vi "Three Ball-Copy (Warning I, Carter did this).vi"() -> ()   [LabVIEW 2014]
uses:
  Team Code/Robot Global Data.vi
panel:
  in  "milliseconds to wait to pull in second ball":u32=1000
  out "Angle":dbl
  out "Distance (in)":dbl
  in  "Min. Power":dbl=0.1 format="%#_13g"
  in  "Roller / Drive Ratio":dbl=1.0
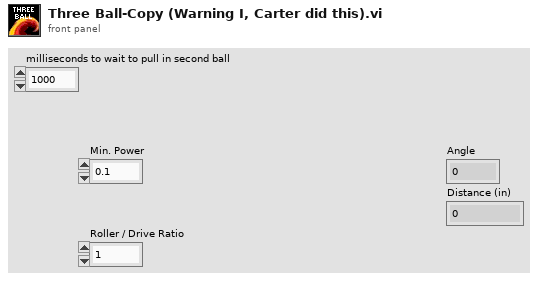
[diagram p1: front panel]
types:
  T1 = cluster{"FIRE!!!":bool, "Loader":bool, "Lock":bool, "Load":bool, "Pass":bool, "Grab":bool, "PANIC":bool, "Don't Cock":bool, "Roller Speed":dbl}
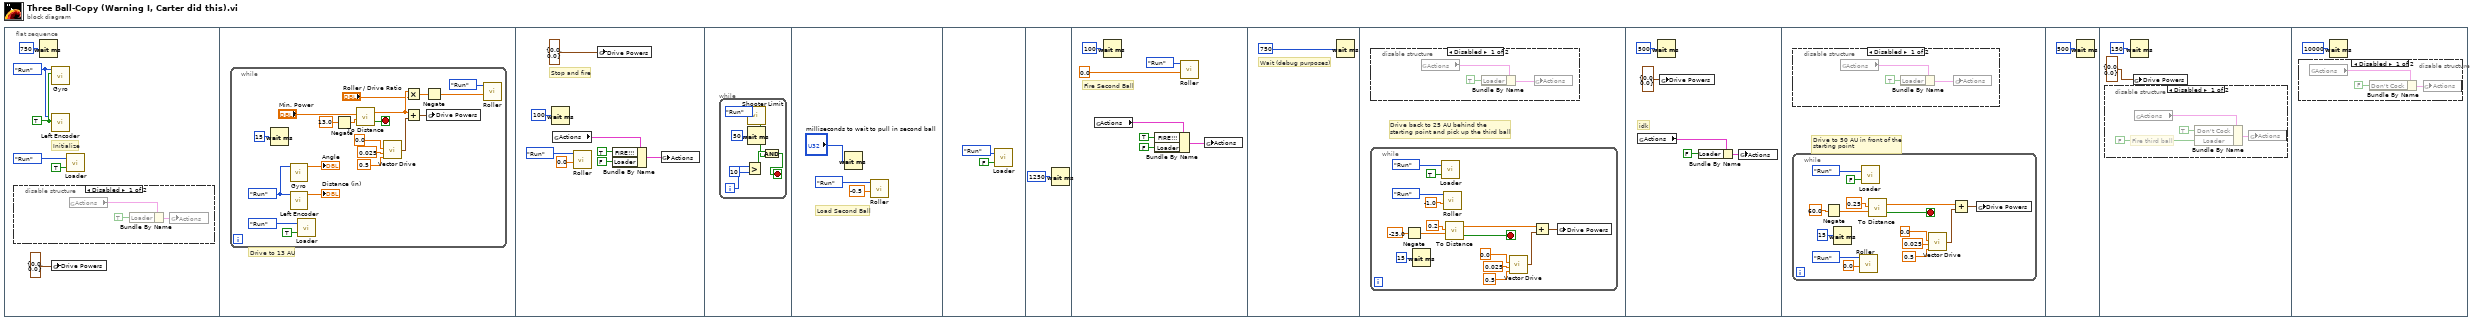
[diagram p0: block diagram]
diagram:
  n1 = flat-sequence {
    frame #0 {
      w5 = enum16{"Start", "Run", "End"}."Run" ("Enum")
      w6 = TRUE ("Reset")
      # "Initialize"
      n2 = disable-structure shown="Disabled" {
        frame Disabled {
          n3 = global read "Robot Global Data.vi" "Actions"() -> (w8:T1)
          n4 = Bundle By Name(cluster=w8, "Loader"=TRUE ("Primary Action")) -> (w9:T1)
          n5 = global write "Robot Global Data.vi" "Actions"(w9) -> ()
        }
        frame Enabled {
        }
      }
      n6 = Wait (ms)(milliseconds to wait=u32 750) -> ()  [unwired: 1 out]
      n7 = call "Gyro.vi"("Reset"=w6, "Enum"=w5) -> ()  [unwired: 9 in, 1 out]
      n8 = call "Left Encoder.vi"("Reset"=w6, "Enum"=w5) -> ()  [unwired: 8 in, 2 out]
      n9 = global write "Robot Global Data.vi" "Drive Powers"(cluster{"Right":dbl, "Left":dbl} {"Right"=0.0, "Left"=0.0} ("Drive Powers")) -> ()
      n10 = call "Loader.vi"("Down (Forward)"=TRUE, "Enum"=enum16{"Start", "Run", "End"}."Run") -> ()  [unwired: 1 out]
    }
    frame #1 {
      # "Drive to 13 AU"
      n11 = while {
        stop <- w28 stop-if-true
        w21 = enum16{"Start", "Run", "End"}."Run" ("Enum")
        n12 = Wait (ms)(milliseconds to wait=u32 15) -> ()  [unwired: 1 out]
        n13 = call "Gyro.vi"("Enum"=w21) -> ("Angle"=→"Angle":dbl)  [unwired: 10 in]
        n14 = call "Left Encoder.vi"("Enum"=w21) -> ("Distance (in)"=→"Distance (in)":dbl)  [unwired: 9 in, 1 out]
        n15 = call "Loader.vi"("Down (Forward)"=TRUE, "Enum"=enum16{"Start", "Run", "End"}."Run") -> ()  [unwired: 1 out]
        n16 = Negate(x=13.0) -> (-x=w19:dbl)
        n17 = call "To Distance.vi"("Destination Dist (in)"=w19, "Min. Power"="Min. Power") -> ("Reached Distance"=w28:bool, "Base Speed"=w17:dbl)  [unwired: 2 in]
        n18 = call "Vector Drive.vi"("Tolerance"=0.5, "Min. Power"=0.025, "Angle"=0.0) -> ("Motor Powers"=w24:cluster{"RMotor":dbl, "LMotor":dbl})  [unwired: 1 in]
        n19 = Multiply(x=w17, y="Roller / Drive Ratio") -> (x*y=w14:dbl)
        n20 = Add(x=w17, y=w24) -> (x+y=w23:cluster{"RMotor":dbl, "LMotor":dbl})
        n21 = Negate(x=w14) -> (-x=w13:dbl)
        n22 = global write "Robot Global Data.vi" "Drive Powers"(w23) -> ()
        n23 = call "Roller.vi"("Power"=w13, "Enum"=enum16{"Start", "Run", "End"}."Run") -> ()  [unwired: 2 in]
      }
    }
    frame #2 {
      # "Stop and fire"
      n24 = Wait (ms)(milliseconds to wait=u32 100) -> ()  [unwired: 1 out]
      n25 = global read "Robot Global Data.vi" "Actions"() -> (w36:T1)
      n26 = call "Roller.vi"("Power"=0.0, "Enum"=enum16{"Start", "Run", "End"}."Run") -> ()  [unwired: 2 in]
      n27 = global write "Robot Global Data.vi" "Drive Powers"(cluster{"Right":dbl, "Left":dbl} {"Right"=0.0, "Left"=0.0} ("Drive Powers")) -> ()
      n28 = Bundle By Name(cluster=w36, "FIRE!!!"=TRUE ("Primary Action"), "Loader"=FALSE) -> (w37:T1)
      n29 = global write "Robot Global Data.vi" "Actions"(w37) -> ()
    }
    frame #3 {
      n30 = while {
        i -> [w42]
        stop <- w38 stop-if-true
        n31 = Greater?(x=w42, y=10) -> (0:w40:bool)
        n32 = call "Shooter Limit.vi"("Enum"=enum16{"Start", "Run", "End"}."Run") -> ("Value"=w39:bool)  [unwired: 1 in]
        n33 = Wait (ms)(milliseconds to wait=u32 50) -> ()  [unwired: 1 out]
        n34 = And(x=w40, y=w39) -> (x .and. y?=w38:bool)
      }
    }
    frame #4 {
      # "Load Second Ball"
      n35 = Wait (ms)(milliseconds to wait="milliseconds to wait to pull in second ball") -> ()  [unwired: 1 out]
      n36 = call "Roller.vi"("Power"=-0.5, "Enum"=enum16{"Start", "Run", "End"}."Run") -> ()  [unwired: 2 in]
    }
    frame #5 {
      n37 = call "Loader.vi"("Down (Forward)"=FALSE, "Enum"=enum16{"Start", "Run", "End"}."Run") -> ()  [unwired: 1 out]
    }
    frame #6 {
      n38 = Wait (ms)(milliseconds to wait=u32 1250) -> ()  [unwired: 1 out]
    }
    frame #7 {
      # "Fire Second Ball"
      n39 = global read "Robot Global Data.vi" "Actions"() -> (w56:T1)
      n40 = Wait (ms)(milliseconds to wait=u32 100) -> ()  [unwired: 1 out]
      n41 = Bundle By Name(cluster=w56, "FIRE!!!"=TRUE ("Primary Action"), "Loader"=FALSE ("Primary Action")) -> (w55:T1)
      n42 = call "Roller.vi"("Power"=0.0, "Enum"=enum16{"Start", "Run", "End"}."Run") -> ()  [unwired: 2 in]
      n43 = global write "Robot Global Data.vi" "Actions"(w55) -> ()
    }
    frame #8 {
      # "Wait (debug purposes)"
      n44 = Wait (ms)(milliseconds to wait=u32 750) -> ()  [unwired: 1 out]
    }
    frame #9 {
      # "Drive back to 25 AU behind the\nstarting point and pick up the third ball"
      n45 = disable-structure shown="Disabled" {
        frame Disabled {
          n46 = global read "Robot Global Data.vi" "Actions"() -> (w60:T1)
          n47 = Bundle By Name(cluster=w60, "Loader"=TRUE) -> (w59:T1)
          n48 = global write "Robot Global Data.vi" "Actions"(w59) -> ()
        }
        frame Enabled {
        }
      }
      n49 = while {
        stop <- w76 stop-if-true
        n50 = Negate(x=-25.0) -> (-x=w70:dbl)
        n51 = Wait (ms)(milliseconds to wait=u32 15) -> ()  [unwired: 1 out]
        n52 = call "Loader.vi"("Down (Forward)"=TRUE, "Enum"=enum16{"Start", "Run", "End"}."Run") -> ()  [unwired: 1 out]
        n53 = call "Roller.vi"("Power"=-1.0, "Enum"=enum16{"Start", "Run", "End"}."Run") -> ()  [unwired: 2 in]
        n54 = call "To Distance.vi"("Destination Dist (in)"=w70, "Min. Power"=0.2) -> ("Reached Distance"=w76:bool, "Base Speed"=w68:dbl)  [unwired: 2 in]
        n55 = call "Vector Drive.vi"("Tolerance"=0.5, "Min. Power"=0.025, "Angle"=0.0) -> ("Motor Powers"=w72:cluster{"RMotor":dbl, "LMotor":dbl})  [unwired: 1 in]
        n56 = Add(x=w68, y=w72) -> (x+y=w71:cluster{"RMotor":dbl, "LMotor":dbl})
        n57 = global write "Robot Global Data.vi" "Drive Powers"(w71) -> ()
      }
    }
    frame #10 {
      # "idk"
      n58 = global read "Robot Global Data.vi" "Actions"() -> (w80:T1)
      n59 = Wait (ms)(milliseconds to wait=u32 500) -> ()  [unwired: 1 out]
      n60 = global write "Robot Global Data.vi" "Drive Powers"(cluster{"Right":dbl, "Left":dbl} {"Right"=0.0, "Left"=0.0} ("Drive Powers")) -> ()
      n61 = Bundle By Name(cluster=w80, "Loader"=FALSE) -> (w81:T1)
      n62 = global write "Robot Global Data.vi" "Actions"(w81) -> ()
    }
    frame #11 {
      # "Drive to 50 AU in front of the\nstarting point"
      n63 = disable-structure shown="Disabled" {
        frame Disabled {
          n64 = global read "Robot Global Data.vi" "Actions"() -> (w83:T1)
          n65 = Bundle By Name(cluster=w83, "Loader"=TRUE) -> (w84:T1)
          n66 = global write "Robot Global Data.vi" "Actions"(w84) -> ()
        }
        frame Enabled {
        }
      }
      n67 = while {
        stop <- w99 stop-if-true
        n68 = Negate(x=60.0) -> (-x=w93:dbl)
        n69 = Wait (ms)(milliseconds to wait=u32 15) -> ()  [unwired: 1 out]
        n70 = call "Roller.vi"("Power"=0.0, "Enum"=enum16{"Start", "Run", "End"}."Run") -> ()  [unwired: 2 in]
        n71 = call "Loader.vi"("Down (Forward)"=FALSE, "Enum"=enum16{"Start", "Run", "End"}."Run") -> ()  [unwired: 1 out]
        n72 = call "To Distance.vi"("Destination Dist (in)"=w93, "Min. Power"=0.25) -> ("Reached Distance"=w99:bool, "Base Speed"=w91:dbl)  [unwired: 2 in]
        n73 = call "Vector Drive.vi"("Tolerance"=0.5, "Min. Power"=0.025, "Angle"=0.0) -> ("Motor Powers"=w95:cluster{"RMotor":dbl, "LMotor":dbl})  [unwired: 1 in]
        n74 = Add(x=w91, y=w95) -> (x+y=w94:cluster{"RMotor":dbl, "LMotor":dbl})
        n75 = global write "Robot Global Data.vi" "Drive Powers"(w94) -> ()
      }
    }
    frame #12 {
      n76 = Wait (ms)(milliseconds to wait=u32 500) -> ()  [unwired: 1 out]
    }
    frame #13 {
      n77 = disable-structure shown="Disabled" {
        frame Disabled {
          # "Fire third ball"
          n78 = global read "Robot Global Data.vi" "Actions"() -> (w106:T1)
          n79 = Bundle By Name(cluster=w106, "Don't Cock"=TRUE ("Primary Action"), "Loader"=FALSE) -> (w105:T1)
          n80 = global write "Robot Global Data.vi" "Actions"(w105) -> ()
        }
        frame Enabled {
        }
      }
      n81 = Wait (ms)(milliseconds to wait=u32 150) -> ()  [unwired: 1 out]
      n82 = global write "Robot Global Data.vi" "Drive Powers"(cluster{"Right":dbl, "Left":dbl} {"Right"=0.0, "Left"=0.0} ("Drive Powers")) -> ()
    }
    frame #14 {
      n83 = disable-structure shown="Disabled" {
        frame Disabled {
          n84 = global read "Robot Global Data.vi" "Actions"() -> (w108:T1)
          n85 = Bundle By Name(cluster=w108, "Don't Cock"=FALSE ("Primary Action")) -> (w109:T1)
          n86 = global write "Robot Global Data.vi" "Actions"(w109) -> ()
        }
        frame Enabled {
        }
      }
      n87 = Wait (ms)(milliseconds to wait=u32 10000) -> ()  [unwired: 1 out]
    }
  }
